vi "Protect Against Broken Encoders.vi"(2 "Rhino Offset":dbl, 3 "Output":dbl) -> (0 "Boolean":bool, 1 "Numeric":dbl)   [LabVIEW 2018]
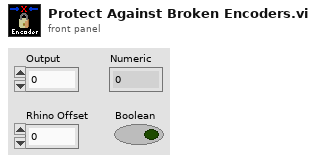
[diagram p1: front panel]
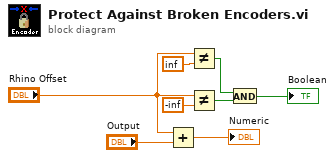
[diagram p0: block diagram]
diagram:
  n1 = Add(x="Rhino Offset", y="Output") -> (x+y=→"Numeric":dbl)
  n2 = Not Equal?(x="Rhino Offset", y=inf) -> (x != y?=w4:bool)
  n3 = Not Equal?(x="Rhino Offset", y=-inf) -> (x != y?=w3:bool)
  n4 = And(x=w4, y=w3) -> (x .and. y?=→"Boolean":bool)
